vi "Find Column Index from Property Value.vi"(7 "Error In":errorcluster, 8 "Channel Property Value":string, 9 "Channel Property Name":string, 10 "Spreadsheet String Array":string[][](array[string])) -> (0 "Error Out":errorcluster, 2 "Column Index":i32, 3 "Spreadsheet String Array Out":string[][](array[string]))   [LabVIEW 2014]
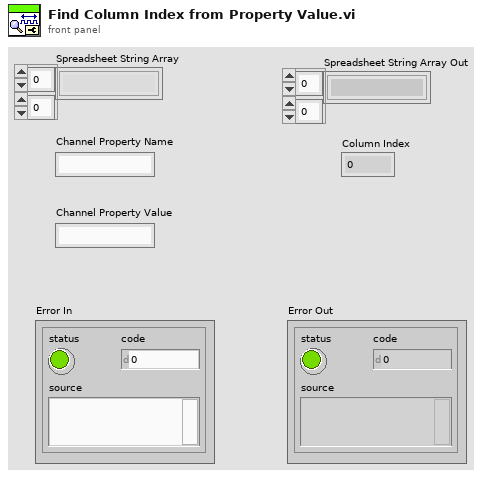
[diagram p1: front panel]
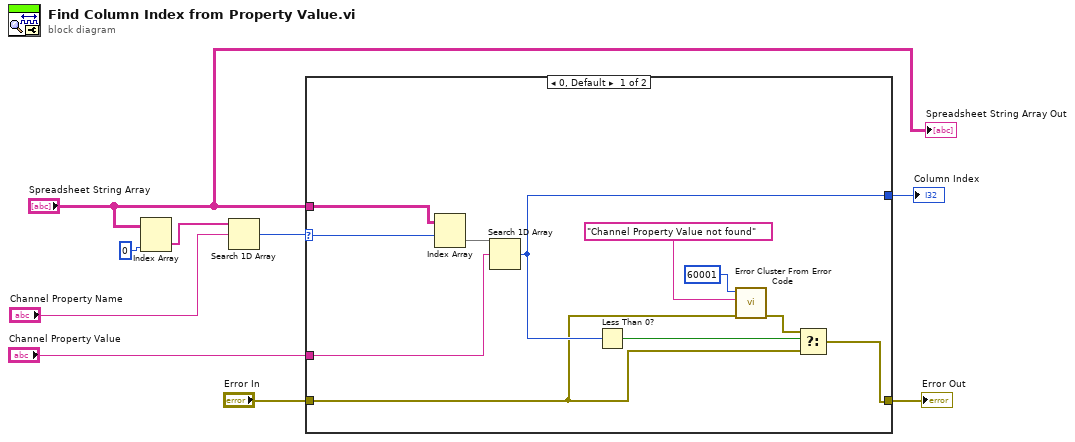
[diagram p0: block diagram]
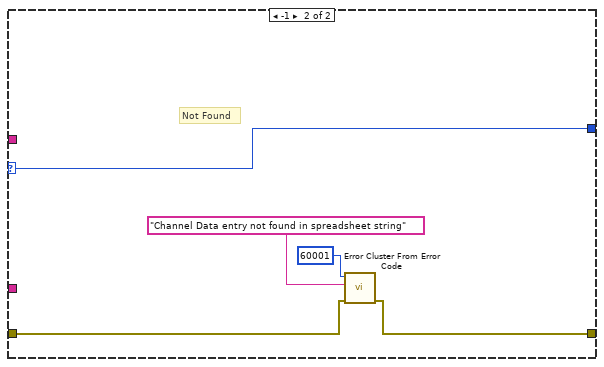
[diagram p2: hidden frame]
diagram:
  n1 = Index Array(array="Spreadsheet String Array", index (col)=0 ("disabled index (col)")) -> (element=w7:string[])  [unwired: 1 in]
  n2 = Search 1D Array(1D array=w7, element="Channel Property Name") -> (index of element=w8:i32)  [unwired: 1 in]
  n3 = case shown="0, Default" w8 {
    selector: w8 -> [w17 w25]
    tunnel: [w16 w25] -> w9
    tunnel: "Error In" -> [w10 w22]
    tunnel: [w11 w21] -> w4
    tunnel: "Channel Property Value" -> [w19 _]
    tunnel: "Spreadsheet String Array" -> [w18 _]
    frame 0, Default {
      n4 = Index Array(array=w18, index (row)=w17) -> (element=w20:string[])  [unwired: 1 in]
      n5 = Search 1D Array(1D array=w20, element=w19) -> (index of element=w16:i32)  [unwired: 1 in]
      n6 = Less Than 0?(x=w16) -> (x < 0?=w15:bool)
      n7 = call <vilib>:"Error Cluster From Error Code.vi"("error in (no error)"=w10, "error message (\"\")"="Channel Property Value not found" ("error message (\"\")"), "error code (0)"=60001) -> ("error out"=w12:errorcluster)  [unwired: 6 in]
      n8 = Select(t=w12, s=w15, f=w10) -> (s? t:f=w11:errorcluster)
    }
    frame -1 {
      # "Not Found"
      n9 = call <vilib>:"Error Cluster From Error Code.vi"("error in (no error)"=w22, "error message (\"\")"="Channel Data entry not found in spreadsheet string" ("error message (\"\")"), "error code (0)"=60001) -> ("error out"=w21:errorcluster)  [unwired: 6 in]
    }
  }
  "Column Index" <- w9
  "Error Out" <- w4
  "Spreadsheet String Array Out" <- "Spreadsheet String Array"
